vi "CAN_Engine(FPGA)_basic.vi"() -> ()   [LabVIEW 2016]
doc: "This example transmits one frame contained in Data Frame every time the Write button is pressed. After building this FPGA VI, you run it using CAN Channel Transmit (Host).vi (not standalone).\n\nThis example assumes the following configuration for CAN 0: Auto Start = True, Listen Only = False, Input Timeout = 10000ms, Output Timeout = 10000ms. The CAN Output node is configured to use an array of U32 for the CAN frame. For more information on configuration, refer to the Help for the NI 9853 CAN module."
uses:
  <vilib>/rvi/Emulation/niFpgaCriticalErrorInLSC.vi
  <vilib>/rvi/Emulation/niFpgaEmulationReportErrorSimple.vi
  <vilib>/rvi/Emulation/niFpgaSctlEmulationGetInTimedLoop.vi
  <vilib>/rvi/Emulation/niFpgaGetClockAttributes.vi
  <vilib>/rvi/Emulation/niFpgaProcessEmulError.vi
  <vilib>/rvi/eio/common/nirviEmuTemplateMethod_errors.vi
  <vilib>/LabVIEW Targets/FPGA/RIO/nicrio_985x_controls.llb/CAN_IO_Frame Array U32.ctl
  <vilib>/eio/EIONode/EIONode.xnode
panel:
  out "U32 In 6":u32
  out "U32 In 5":u32
  out "U32 In 4":u32
  out "U32 In 3":u32
  out "U32 In 2":u32
  in  "Write":bool
  in  "U32 Out 6":u32
  in  "U32 Out 5":u32
  in  "U32 Out 4":u32
  in  "U32 Out 3":u32
  in  "Ready":bool
  out "U32 In":u32
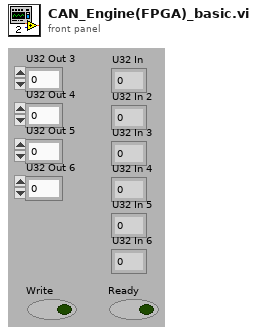
[diagram p1: front panel]
types:
  T1 = typedef "CAN_IO_Frame Array U32.ctl" = u32[]
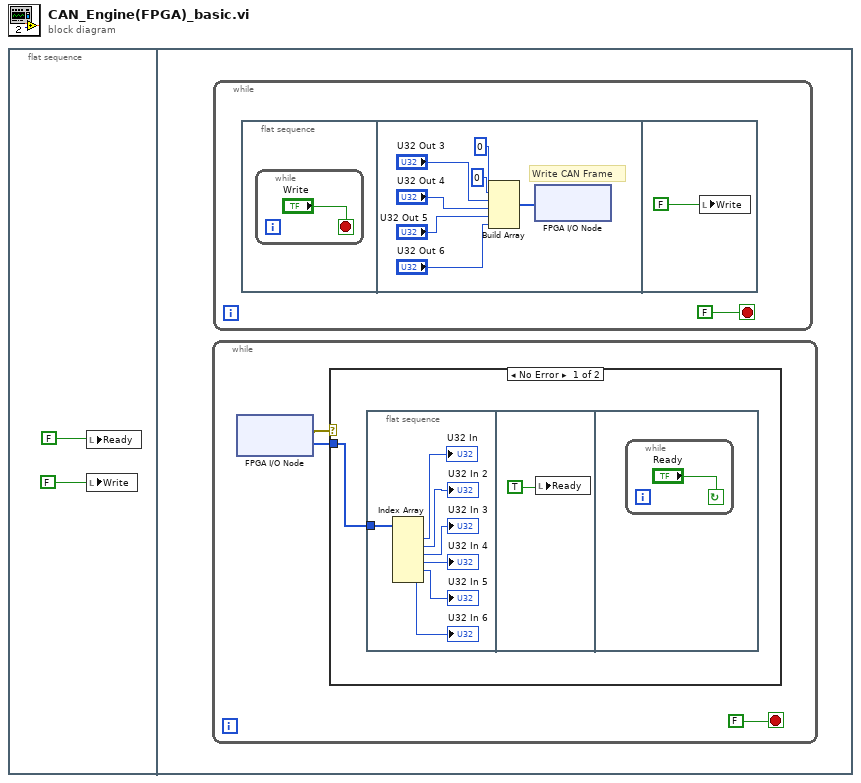
[diagram p0: block diagram]
diagram:
  n1 = flat-sequence {
    frame #0 {
      n2 = local write "Ready"(FALSE) -> ()
      n3 = local write "Write"(FALSE ("Write")) -> ()
    }
    frame #1 {
      n4 = while {
        stop <- FALSE stop-if-true
        n5 = xnode "FPGA I/O Node"() -> ("error out"=w5:errorcluster, "CAN0"=w4:T1)  [unwired: 2 in, 1 out]
        n6 = case shown="No Error" w5 {
          tunnel: w4 -> [w6 _]
          frame No Error {
            n7 = flat-sequence {
              tunnel: w6 -> [w7]
              frame #0 {
                n8 = Index Array(array=w7) -> (element #1=→"U32 In":u32, element #2=→"U32 In 2":u32, element #3=→"U32 In 3":u32, element #4=→"U32 In 4":u32, element #5=→"U32 In 5":u32, element #6=→"U32 In 6":u32)  [unwired: 6 in]
              }
              frame #1 {
                n9 = local write "Ready"(TRUE ("Ready")) -> ()
              }
              frame #2 {
                n10 = while {
                  stop <- "Ready" continue-if-true
                }
              }
            }
          }
          frame Error {
          }
        }
      }
      n11 = while {
        stop <- FALSE stop-if-true
        n12 = flat-sequence {
          frame #0 {
            n13 = while {
              stop <- "Write" stop-if-true
            }
          }
          frame #1 {
            # "Write CAN Frame"
            n14 = Build Array(u32 0 ("element"), u32 0 ("element"), "U32 Out 3", "U32 Out 4", "U32 Out 5", "U32 Out 6") -> (w18:u32[])
            n15 = xnode "FPGA I/O Node"("CAN0"=w18) -> ()  [unwired: 1 in, 1 out]
          }
          frame #2 {
            n16 = local write "Write"(FALSE ("Write")) -> ()
          }
        }
      }
    }
  }
